vi "Compute V50.vi"(5 "Partial":sgl[](array[numeric]) format="%.2f", 6 "Maximum Deviation":sgl format="%.2f", 7 "Complete":sgl[](array[numeric]) format="%.2f") -> (0 "velSTDEV":sgl caption="Standard Deviation" min=0 max=10000 step=1 format="%.1f", 1 "Pairs":i16, 2 "zmr":sgl format="%.2f", 3 "V50":sgl format="%.2f")   [LabVIEW 2015]
uses:
  <vilib>/Analysis/NI_AALBase.lvlib
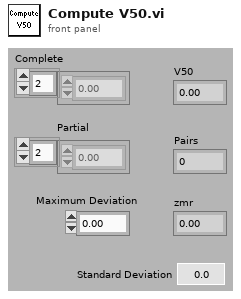
[diagram p1: front panel]
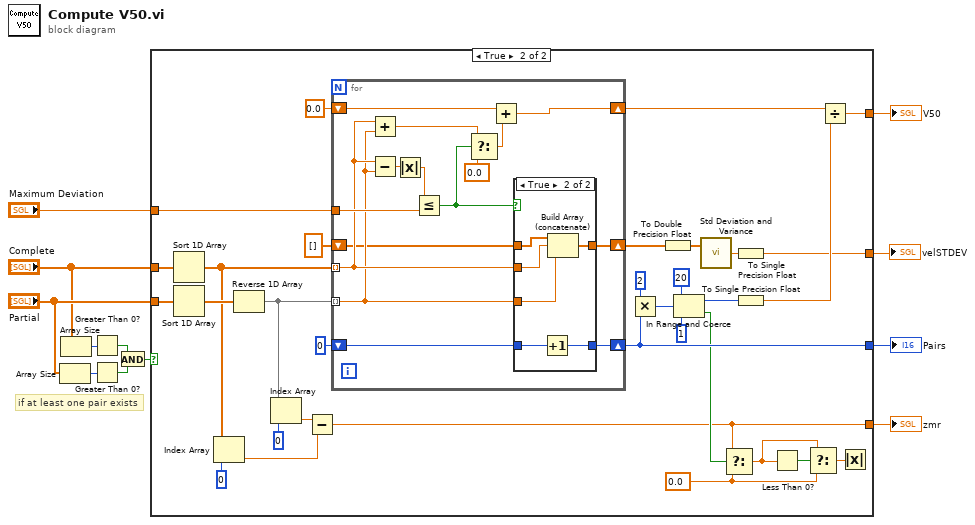
[diagram p0: block diagram]
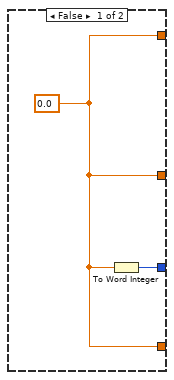
[diagram p2: hidden frame]
diagram:
  # "if at least one pair exists"
  n1 = Array Size(array="Partial") -> (size(s)=w7:i32)
  n2 = Array Size(array="Complete") -> (size(s)=w6:i32)
  n3 = Greater Than 0?(x=w6) -> (x > 0?=w5:bool)
  n4 = Greater Than 0?(x=w7) -> (x > 0?=w4:bool)
  n5 = And(x=w5, y=w4) -> (x .and. y?=w3:bool)
  n6 = case shown="True" w3 {
    tunnel: [w14 w41] -> w8
    tunnel: [w13 w29] -> w9
    tunnel: "Complete" -> [_ w37]
    tunnel: "Partial" -> [_ w36]
    tunnel: "Maximum Deviation" -> [_ w35]
    tunnel: [w14 w23] -> w2
    tunnel: [w14 w15] -> w1
    frame False {
      w14 = sgl 0.0
      n7 = To Word Integer(number=w14) -> (16bit integer=w13:i16)
    }
    frame True {
      w26 = sgl 0.0 ("f")
      n8 = Sort 1D Array(array=w37) -> (sorted array=w31:sgl[])
      n9 = Sort 1D Array(array=w36) -> (sorted array=w46:sgl[])
      n10 = Index Array(array=w31, index=0 ("Index")) -> (element=w21:sgl)
      n11 = Reverse 1D Array(array=w46) -> (reversed array=w32:sgl[])
      n12 = Index Array(array=w32, index=0 ("Index")) -> (element=w22:sgl)
      n13 = Subtract(x=w22, y=w21) -> (x-y=w23:sgl)
      n14 = for {
        shift-right: [w60] -> w42
        shift-left: sgl 0.0 -> [w59]
        tunnel: w32 -> [w49] mode=indexing
        tunnel: w31 -> [w50] mode=indexing
        shift-right: [w54] -> w29
        shift-left: i16 0 -> [w55]
        tunnel: w35 -> [w52]
        shift-right: [w48] -> w16
        shift-left: sgl[] [] -> [w47]
        n15 = Add(x=w50, y=w49) -> (x+y=w57:sgl)
        n16 = Subtract(x=w50, y=w49) -> (x-y=w61:sgl)
        n17 = Absolute Value(x=w61) -> (abs(x)=w53:sgl)
        n18 = Less Or Equal?(x=w53, y=w52) -> (x <= y?=w56:bool)
        n19 = Select(t=w57, s=w56, f=sgl 0.0) -> (s? t:f=w51:sgl)
        n20 = Add(x=w59, y=w51) -> (x+y=w60:sgl)
        n21 = case shown="True" w56 {
          tunnel: w55 -> [w63 w69]
          tunnel: [w63 w68] -> w54
          tunnel: w50 -> [_ w67]
          tunnel: w49 -> [_ w66]
          tunnel: [w62 w65] -> w48
          tunnel: w47 -> [w62 w64]
          frame False {
          }
          frame True {
            n22 = Increment(x=w69) -> (x+1=w68:i16)
            n23 = Build Array (concatenate)(w64, w67, w66) -> (w65:sgl[])
          }
        }
      }
      n24 = Multiply(x=i16 2, y=w29) -> (x*y=w38:i16)
      n25 = To Double Precision Float(number=w16) -> (double precision float=w18:dbl[])
      n26 = In Range and Coerce(upper limit=i16 20, x=w38, lower limit=i16 1) -> (coerced(x)=w34:i16, In Range?=w28:bool)
      n27 = call <vilib>:"Std Deviation and Variance.vi"("X"=w18) -> ("standard deviation"=w17:dbl)  [unwired: 1 in, 2 out]
      n28 = Select(t=w23, s=w28, f=w26) -> (s? t:f=w24:sgl)
      n29 = To Single Precision Float(number=w17) -> (single precision float=w15:sgl)
      n30 = To Single Precision Float(number=w34) -> (single precision float=w20:sgl)
      n31 = Less Than 0?(x=w24) -> (x < 0?=w27:bool)
      n32 = Select(t=w24, s=w27, f=w26) -> (s? t:f=w25:sgl)
      n33 = Divide(x=w42, y=w20) -> (x/y=w41:sgl)
      n34 = Absolute Value(x=w25) -> ()  [unwired: 1 out]
    }
  }
  "Pairs" <- w9
  "V50" <- w8
  "zmr" <- w2
  "velSTDEV" <- w1
